vi "EventServer_ClientUnhandledEvents.vi"(8 "error in (no error)":errorcluster, 11 "Client Name":string) -> (0 "error out":errorcluster, 3 "Subscription":string[](array[string]))   [LabVIEW 2011]
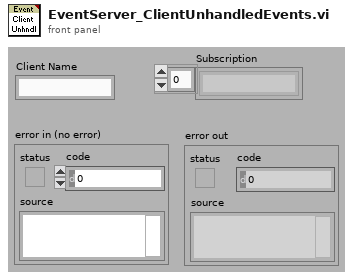
[diagram p1: front panel]
types:
  T1 = cluster{"Client":refnum<queue>, "Sub Events":string[], "PrvData":variant, "MyName":string}
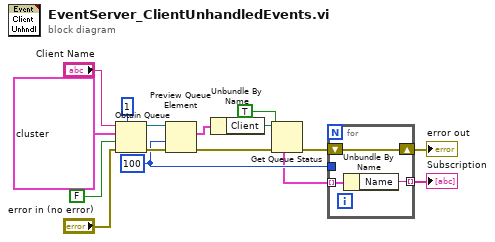
[diagram p0: block diagram]
diagram:
  w3 = 100 ("timeout in ms (-1)")
  n1 = Obtain Queue(max queue size (-1, unlimited)=1, name (unnamed)="Client Name", element data type=T1 {"Client"=refnum, "Sub Events"=[], "PrvData"=variant, "MyName"=""} ("output cluster"), create if not found? (T)=FALSE, error in (no error)="error in (no error)") -> (queue out=w12:refnum<queue>, error out=w11:errorcluster)  [unwired: 1 out]
  n2 = Preview Queue Element(queue=w12, timeout in ms (-1)=w3, error in (no error)=w11) -> (element=w10:T1, error out=w7:errorcluster)  [unwired: 2 out]
  n3 = Unbundle By Name(w10) -> ("Client"=w8:refnum<queue>)
  n4 = Get Queue Status(queue=w8, return elements? (F)=TRUE, error in (no error)=w7) -> (error out=w6:errorcluster, elements=w2:cluster{"Name":string, "Data":variant}[])  [unwired: 6 out]
  n5 = for {
    shift-right: [w17] -> w5
    shift-left: w6 -> [w17]
    tunnel: [w19] -> w4 mode=indexing
    tunnel: w3 -> [_]
    tunnel: w2 -> [w18] mode=indexing
    n6 = Unbundle By Name(w18) -> ("Name"=w19:string)
  }
  "error out" <- w5
  "Subscription" <- w4
